vi "System-User-Async-Host.vi"() -> ()   [LabVIEW 2016]
uses:
  Shared/Typedefs/UserParameter-Array.ctl
  Shared/Typedefs/UserParameter.ctl
  Shared/DSI-Shared.lvlib
panel:
  in  "_Label":string caption="User Plugin (Asynchronous)"
  in  "Enable":bool
  in  "Filename":string caption="User VI File Path (.vi relative to default data directory)"
  in  "dt":sgl caption="[ms]"
  out "Error":bool caption="User VI Error"
  in  "Reload":bool
  in  "_User Param":string[][](table) caption="User Parameters"
  in  "_Hidden":enum32{"Page 1"}(tab)
  out "SYS|User|ParamNames":string[](array[string])
  in  "SYS|User|ParamValues":sgl[](array[numeric])
  out "SYS|User|Results":T1=[{"Name"="", "Value"=0.0}, {"Name"="", "Value"=0.0}, {"Name"="", "Value"=0.0}, {"Name"="", "Value"=0.0}, {"Name"="", "Value"=0.0}, {"Name"="", "Value"=0.0}, {"Name"="", "Value"=0.0}, {"Name"="", "Value"=0.0}, {"Name"="", "Value"=0.0}, {"Name"="", "Value"=0.0}, {"Name"="", "Value"=0.0}, {"Name"="", "Value"=0.0}, {"Name"="", "Value"=0.0}, {"Name"="", "Value"=0.0}, {"Name"="", "Value"=0.0}, {"Name"="", "Value"=0.0}, {"Name"="", "Value"=0.0}, {"Name"="", "Value"=0.0}, {"Name"="", "Value"=0.0}, {"Name"="", "Value"=0.0}, {"Name"="", "Value"=0.0}, {"Name"="", "Value"=0.0}, {"Name"="", "Value"=0.0}, {"Name"="", "Value"=0.0}, {"Name"="", "Value"=0.0}, {"Name"="", "Value"=0.0}, {"Name"="", "Value"=0.0}, {"Name"="", "Value"=0.0}, {"Name"="", "Value"=0.0}, {"Name"="", "Value"=0.0}, {"Name"="", "Value"=0.0}, {"Name"="", "Value"=0.0}, {"Name"="", "Value"=0.0}, {"Name"="", "Value"=0.0}, {"Name"="", "Value"=0.0}, {"Name"="", "Value"=0.0}, {"Name"="", "Value"=0.0}, {"Name"="", "Value"=0.0}, {"Name"="", "Value"=0.0}, {"Name"="", "Value"=0.0}, {"Name"="", "Value"=0.0}, {"Name"="", "Value"=0.0}, {"Name"="", "Value"=0.0}, {"Name"="", "Value"=0.0}, {"Name"="", "Value"=0.0}, {"Name"="", "Value"=0.0}, {"Name"="", "Value"=0.0}, {"Name"="", "Value"=0.0}, {"Name"="", "Value"=0.0}, {"Name"="", "Value"=0.0}, {"Name"="", "Value"=0.0}, {"Name"="", "Value"=0.0}, {"Name"="", "Value"=0.0}, {"Name"="", "Value"=0.0}, {"Name"="", "Value"=0.0}, {"Name"="", "Value"=0.0}, {"Name"="", "Value"=0.0}, {"Name"="", "Value"=0.0}, {"Name"="", "Value"=0.0}, {"Name"="", "Value"=0.0}, {"Name"="", "Value"=0.0}, {"Name"="", "Value"=0.0}, {"Name"="", "Value"=0.0}, {"Name"="", "Value"=0.0}, {"Name"="", "Value"=0.0}, {"Name"="", "Value"=0.0}, {"Name"="", "Value"=0.0}, {"Name"="", "Value"=0.0}, {"Name"="", "Value"=0.0}, {"Name"="", "Value"=0.0}, {"Name"="", "Value"=0.0}, {"Name"="", "Value"=0.0}, {"Name"="", "Value"=0.0}, {"Name"="", "Value"=0.0}, {"Name"="", "Value"=0.0}, {"Name"="", "Value"=0.0}, {"Name"="", "Value"=0.0}, {"Name"="", "Value"=0.0}, {"Name"="", "Value"=0.0}, {"Name"="", "Value"=0.0}, {"Name"="", "Value"=0.0}, {"Name"="", "Value"=0.0}, {"Name"="", "Value"=0.0}, {"Name"="", "Value"=0.0}, {"Name"="", "Value"=0.0}, {"Name"="", "Value"=0.0}, {"Name"="", "Value"=0.0}, {"Name"="", "Value"=0.0}, {"Name"="", "Value"=0.0}, {"Name"="", "Value"=0.0}, {"Name"="", "Value"=0.0}, {"Name"="", "Value"=0.0}, {"Name"="", "Value"=0.0}, {"Name"="", "Value"=0.0}, {"Name"="", "Value"=0.0}, {"Name"="", "Value"=0.0}, {"Name"="", "Value"=0.0}, {"Name"="", "Value"=0.0}, {"Name"="", "Value"=0.0}, {"Name"=" ", "Value"=0.0}]
  out "_User Results":string[][](table) caption="User Results"
  # "Enable Plugin"
  # "File Path (.lvclass relative to default data directory)"
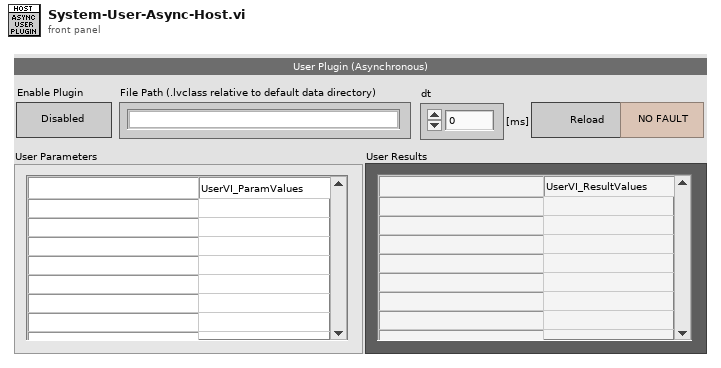
[diagram p1: front panel]
types:
  T1 = typedef "DSI-Shared.lvlib/UserParameter-Array.ctl" = T2[]
  T2 = typedef "DSI-Shared.lvlib/UserParameter.ctl" = cluster{"Name":string, "Value":dbl}
  T3 = typedef "LVBoundsTypeDef.ctl" = cluster{"Width":u32, "Height":u32}
  T4 = typedef "LVRectTypeDef.ctl" = cluster{"Left":i16, "Top":i16, "Right":i16, "Bottom":i16}
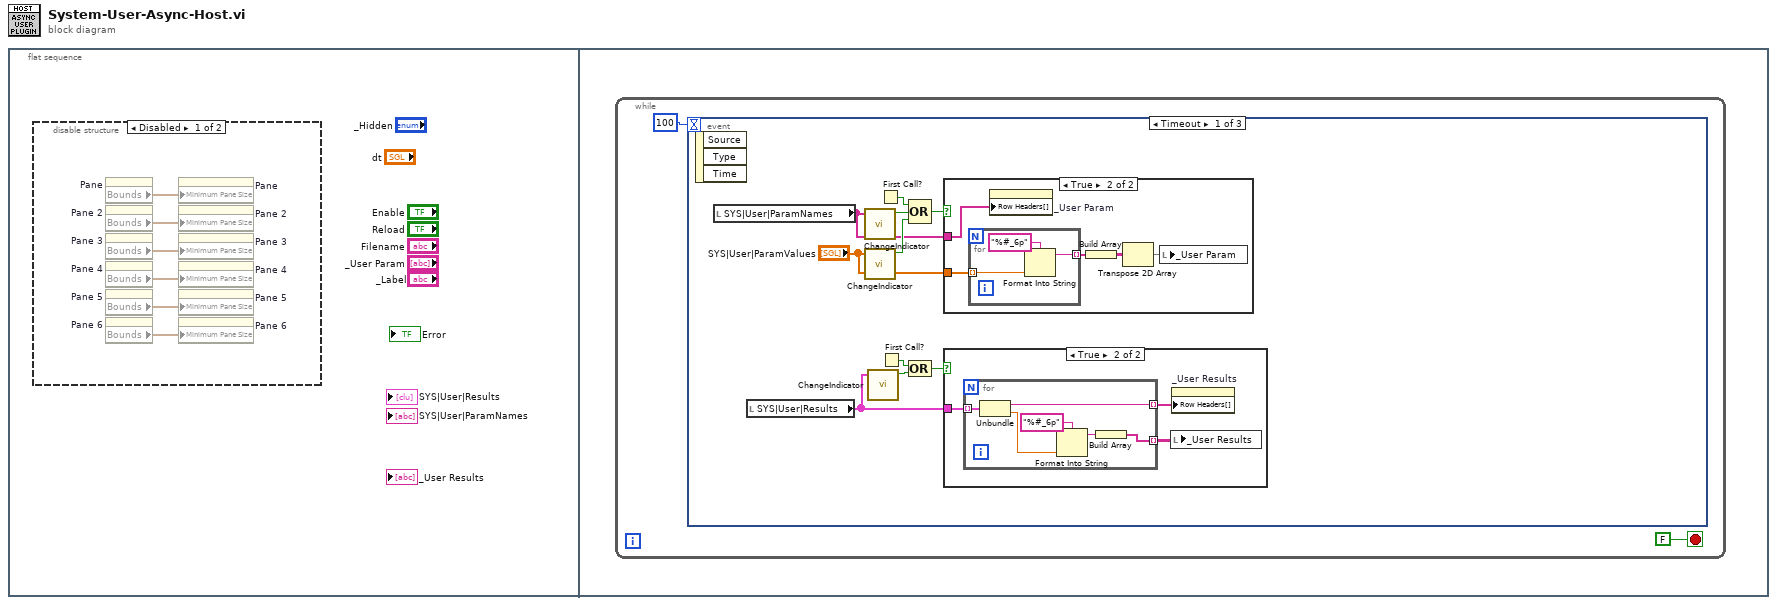
[diagram p0: block diagram]
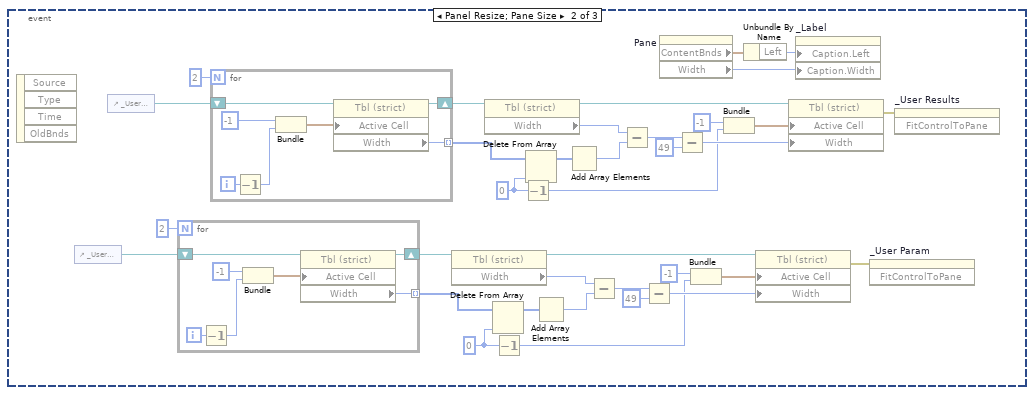
[diagram p5: hidden frame]
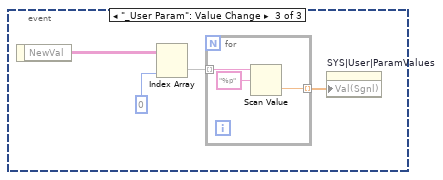
[diagram p6: hidden frame]
diagram:
  n1 = flat-sequence {
    frame #0 {
      n2 = disable-structure shown="Disabled" {
        frame Disabled {
          n3 = property on="Pane" class="Pane"() -> ("Bounds"=w6:T3)  [unwired: 2 in, 2 out]
          n4 = property on="Pane 2" class="Pane"() -> ("Bounds"=w5:T3)  [unwired: 2 in, 2 out]
          n5 = property on="Pane 3" class="Pane"() -> ("Bounds"=w4:T3)  [unwired: 2 in, 2 out]
          n6 = property on="Pane 4" class="Pane"() -> ("Bounds"=w3:T3)  [unwired: 2 in, 2 out]
          n7 = property on="Pane 5" class="Pane"() -> ("Bounds"=w2:T3)  [unwired: 2 in, 2 out]
          n8 = property on="Pane 6" class="Pane"() -> ("Bounds"=w1:T3)  [unwired: 2 in, 2 out]
          n9 = property on="Pane" class="Pane"("Minimum Pane Size"=w6) -> ()  [unwired: 2 in, 2 out]
          n10 = property on="Pane 2" class="Pane"("Minimum Pane Size"=w5) -> ()  [unwired: 2 in, 2 out]
          n11 = property on="Pane 3" class="Pane"("Minimum Pane Size"=w4) -> ()  [unwired: 2 in, 2 out]
          n12 = property on="Pane 4" class="Pane"("Minimum Pane Size"=w3) -> ()  [unwired: 2 in, 2 out]
          n13 = property on="Pane 5" class="Pane"("Minimum Pane Size"=w2) -> ()  [unwired: 2 in, 2 out]
          n14 = property on="Pane 6" class="Pane"("Minimum Pane Size"=w1) -> ()  [unwired: 2 in, 2 out]
        }
        frame Enabled {
        }
      }
    }
    frame #1 {
      n15 = while {
        stop <- FALSE stop-if-true
        n16 = event shown="[0] Timeout" {
          selector: _ -> [_ _ _]
          dyn-events: _ -> [_ _ _]
          timeout: 100 ("millisecond multiple") -> [_ _ _]
          event Timeout {
            n17 = event-data() -> ()  [unwired: 1 in, 3 out]
            n18 = local read "SYS|User|ParamNames"() -> (w11:string[])
            n19 = local read "SYS|User|Results"() -> (w10:T1)
            n20 = call "ChangeIndicator.vi"("Input"=w11) -> ("Change"=w16:bool)  [unwired: 9 in]
            n21 = call "ChangeIndicator.vi"("Input"="SYS|User|ParamValues") -> ("Change"=w15:bool)  [unwired: 9 in]
            n22 = call "ChangeIndicator.vi"("Input"=w10) -> ("Change"=w13:bool)  [unwired: 9 in]
            n23 = First Call?() -> (First Call?: T/F=w12:bool)
            n24 = First Call?() -> (First Call?: T/F=w9:bool)
            n25 = Compound Arithmetic op=OR(w12, w16, w15) -> (w14:bool)
            n26 = Compound Arithmetic op=OR(w9, w13) -> (w18:bool)
            n27 = case shown="True" w14 {
              tunnel: "SYS|User|ParamValues" -> [_ w19]
              tunnel: w11 -> [_ w21]
              frame False {
              }
              frame True {
                n28 = for {
                  tunnel: w19 -> [w26] mode=indexing
                  tunnel: [w25] -> w20 mode=indexing
                  n29 = Format Into String(format string="%#_6p", w26) -> (resulting string=w25:string)  [unwired: 2 in, 1 out]
                }
                n30 = property on="_User Param" class="Tbl (strict)"("Row Headers[]"=w21) -> ()  [unwired: 2 in, 2 out]
                n31 = Build Array(w20) -> (w23:string[][])
                n32 = Transpose 2D Array(2D array=w23) -> (transposed array=w22:string[][])
                n33 = local write "_User Param"(w22) -> ()
              }
            }
            n34 = case shown="True" w18 {
              tunnel: w10 -> [_ w29]
              frame False {
              }
              frame True {
                n35 = for {
                  tunnel: [w33] -> w27 mode=indexing
                  tunnel: w29 -> [w35] mode=indexing
                  tunnel: [w34] -> w28 mode=indexing
                  n36 = Unbundle(w35) -> ("Name"=w34:string, "Value"=w30:dbl)
                  n37 = Format Into String(format string="%#_6p", w30) -> (resulting string=w31:string)  [unwired: 2 in, 1 out]
                  n38 = Build Array(w31) -> (w33:string[])
                }
                n39 = local write "_User Results"(w27) -> ()
                n40 = property on="_User Results" class="Tbl (strict)"("Row Headers[]"=w28) -> ()  [unwired: 2 in, 2 out]
              }
            }
          }
          event Panel Resize; Pane Size {
            w47 = 0 ("index")
            w65 = 0 ("index")
            n41 = event-data() -> ()  [unwired: 1 in, 4 out]
            n42 = control-ref of="_User Param"() -> (w69:refnum<vi>)
            n43 = control-ref of="_User Results"() -> (w43:refnum<vi>)
            n44 = for {
              N: 2 -> [_]
              shift-right: [w81] -> w60
              shift-left: w69 -> [w82]
              tunnel: [w79] -> w61 mode=indexing
              i -> [w84]
              n45 = Decrement(x=w84) -> (x-1=w78:i32)
              n46 = Bundle(-1, w78) -> (w80:cluster{i32, i32})  [unwired: 1 in]
              n47 = property class="Tbl (strict)"(reference=w82, "Active Cell"=w80) -> (reference out=w81:refnum<vi>, "Width"=w79:u32)  [unwired: 1 in, 1 out]
            }
            n48 = for {
              N: 2 -> [_]
              shift-right: [w74] -> w52
              shift-left: w43 -> [w75]
              tunnel: [w72] -> w51 mode=indexing
              i -> [w77]
              n49 = Decrement(x=w77) -> (x-1=w71:i32)
              n50 = Bundle(-1, w71) -> (w73:cluster{i32, i32})  [unwired: 1 in]
              n51 = property class="Tbl (strict)"(reference=w75, "Active Cell"=w73) -> (reference out=w74:refnum<vi>, "Width"=w72:u32)  [unwired: 1 in, 1 out]
            }
            n52 = property on="Property Node" class="Tbl (strict)"(reference=w60) -> (reference out=w59:refnum<vi>, "Width"=w58:u32)  [unwired: 1 in, 1 out]
            n53 = property on="Property Node" class="Tbl (strict)"(reference=w52) -> (reference out=w53:refnum<vi>, "Width"=w54:u32)  [unwired: 1 in, 1 out]
            n54 = Delete From Array(array=w61, index=w65) -> (array with subset deleted=w62:u32[])  [unwired: 1 in, 1 out]
            n55 = Decrement(x=w65) -> (x-1=w56:i32)
            n56 = Decrement(x=w47) -> (x-1=w41:i32)
            n57 = Delete From Array(array=w51, index=w47) -> (array with subset deleted=w50:u32[])  [unwired: 1 in, 1 out]
            n58 = Add Array Elements(numeric array=w62) -> (sum=w63:u32)
            n59 = Add Array Elements(numeric array=w50) -> (sum=w49:u32)
            n60 = Subtract(x=w58, y=w63) -> (x-y=w57:u32)
            n61 = Subtract(x=w54, y=w49) -> (x-y=w55:u32)
            n62 = Subtract(x=w57, y=u32 49) -> (x-y=w67:u32)
            n63 = property on="Pane" class="Pane"() -> ("ContentBnds"=w39:T4, "Width"=w40:u32)  [unwired: 2 in, 2 out]
            n64 = Subtract(x=w55, y=u32 49) -> (x-y=w45:u32)
            n65 = Bundle(-1, w56) -> (w66:cluster{i32, i32})  [unwired: 1 in]
            n66 = Bundle(-1, w41) -> (w46:cluster{i32, i32})  [unwired: 1 in]
            n67 = Unbundle By Name(w39) -> ("Left"=w38:i16)
            n68 = property on="Property Node" class="Tbl (strict)"(reference=w59, "Active Cell"=w66, "Width"=w67) -> (error out=w36:errorcluster)  [unwired: 1 in, 1 out]
            n69 = property on="Property Node" class="Tbl (strict)"(reference=w53, "Active Cell"=w46, "Width"=w45) -> (error out=w37:errorcluster)  [unwired: 1 in, 1 out]
            n70 = property on="_Label" class="Str"("Caption.Left"=w38, "Caption.Width"=w40) -> ()  [unwired: 2 in, 2 out]
            n71 = invoke on="_User Param" class="Tbl (strict)" method="FitControlToPane"(error in=w36) -> ()  [unwired: 2 in, 3 out]
            n72 = invoke on="_User Results" class="Tbl (strict)" method="FitControlToPane"(error in=w37) -> ()  [unwired: 2 in, 3 out]
          }
          event "_User Param": Value Change {
            n73 = event-data() -> ("NewVal"=w88:string[][])  [unwired: 1 in]
            n74 = Index Array(array=w88, index (col)=0 ("disabled index (col)")) -> (element=w86:string[])  [unwired: 1 in]
            n75 = for {
              tunnel: [w91] -> w85 mode=indexing
              tunnel: w86 -> [w90] mode=indexing
              n76 = Scan Value(string=w90, format string="%p") -> (value=w91:dbl)  [unwired: 1 in, 1 out]
            }
            n77 = property on="SYS|User|ParamValues" class="Arr (strict)"("Val(Sgnl)"=w85) -> ()  [unwired: 2 in, 2 out]
          }
        }
      }
    }
  }
